vi "test FXP Write and Read.vi"(8 "error in (no error)":errorcluster, 11 "Scalar Channels Testing in":refnum<class "FPGA Addon Scalar Channels System Tests.lvclass">) -> (0 "error out":errorcluster, 3 "Scalar Channels Testing out":refnum<class "FPGA Addon Scalar Channels System Tests.lvclass">)   [LabVIEW 2018, in "FPGA Addon Scalar Channels System Tests.lvclass"]
uses:
  FPGA Addon Scalar Channels System Tests.lvclass
  C:/Dev/niveristand-fpga-addon-custom-device-1/Source/Tests/FPGA Addon Test Class/FPGA Addon Test Class.lvclass
  C:/Program Files (x86)/National Instruments/LabVIEW 2018/vi.lib/NI/NI VS CD Testing Tools/VeriStandTestCase/VeriStandTestCase.lvclass
  FPGA Addon Test Class/FPGA Addon Test Class.lvclass/FPGA Addon Test Class.ctl
  FPGA Addon Test Class/FPGA Addon Test Class.lvclass
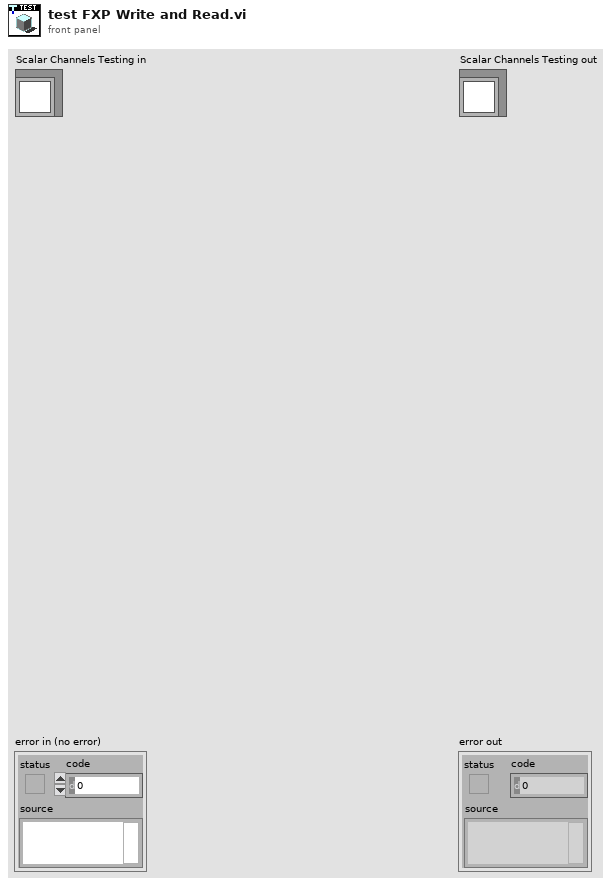
[diagram p1: front panel]
types:
  T1 = typedef "NI_VS Workspace ExecutionAPI.lvlib/WorkspaceAPI.ctl" = refnum<k24>
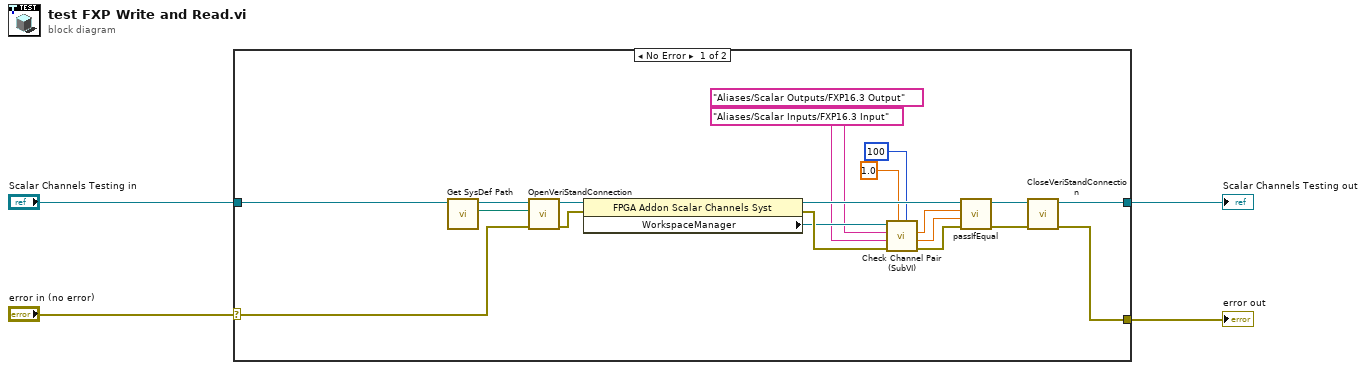
[diagram p0: block diagram]
diagram:
  n1 = case shown="No Error" "error in (no error)" {
    selector: "error in (no error)" -> [w17 w26]
    tunnel: [w23 w26] -> w3
    tunnel: [w24 w25] -> w1
    tunnel: "Scalar Channels Testing in" -> [w16 w25]
    frame No Error {
      n2 = call "Get SysDef Path.vi"("Scalar Channels Testing in"=w16) -> ("SysDef Path"=w14:path, "Scalar Channels Testing out"=w15:refnum<class "FPGA Addon Scalar Channels System Tests.lvclass">)  [unwired: 9 in]
      n3 = call-dynamic "OpenVeriStandConnection.vi"("error in (no error)"=w17, "System Definition File"=w14, "VeriStand Test Case in"=w15) -> ("error out"=w22:errorcluster, "VeriStand Test Case out"=w21:refnum<class "FPGA Addon Scalar Channels System Tests.lvclass">)  [unwired: 6 in, 1 out]
      n4 = property class="FPGA Addon Scalar Channels Syst"(reference=w21, error in=w22) -> (reference out=w20:refnum<class "FPGA Addon Scalar Channels System Tests.lvclass">, error out=w13:errorcluster, "WorkspaceManager"=w10:T1)
      n5 = call "Check Channel Pair (SubVI).vi"("milliseconds to wait"=u32 100, "Test Value"=1.0 ("Value"), "error in (no error)"=w13, "Input Channel"="Aliases/Scalar Inputs/FXP16.3 Input" ("Channel"), "Output Channel"="Aliases/Scalar Outputs/FXP16.3 Output" ("Channel"), "WorkspaceManager in"=w10) -> ("error out"=w5:errorcluster, "InputChannel Value"=w6:dbl, "OutputChannel Value"=w7:dbl)  [unwired: 2 in, 1 out]
      n6 = call-dynamic "passIfEqual.vi"("error in (no error)"=w5, "y"=w6, "x"=w7, "TestCase in"=w20) -> ("error out"=w18:errorcluster, "TestCase out"=w19:refnum<class "FPGA Addon Scalar Channels System Tests.lvclass">)  [unwired: 6 in]
      n7 = call-dynamic "CloseVeriStandConnection.vi"("error in (no error)"=w18, "VeriStand Test Case in"=w19) -> ("error out"=w23:errorcluster, "VeriStand Test Case out"=w24:refnum<class "FPGA Addon Scalar Channels System Tests.lvclass">)  [unwired: 8 in]
    }
    frame Error {
    }
  }
  "error out" <- w3
  "Scalar Channels Testing out" <- w1
